vi "spindle_speed_1.vi"(0 "Byte Stream File in":refnum<file>, 2 "Array":dbl[](array[numeric]), 5 "base path":path, 7 "Record  SS 661":bool, 9 "Boolean 3":bool, 11 "error in (no error)":errorcluster, 12 "Initial Time in":timestamp, 13 "Stop Program 4":bool) -> (4 "Byte Stream File out":refnum<file>, 6 "Boolean 2":bool, 8 "Initial Time out":timestamp, 10 "Stop Program 5":bool, 15 "error out":errorcluster)   [LabVIEW 2014]
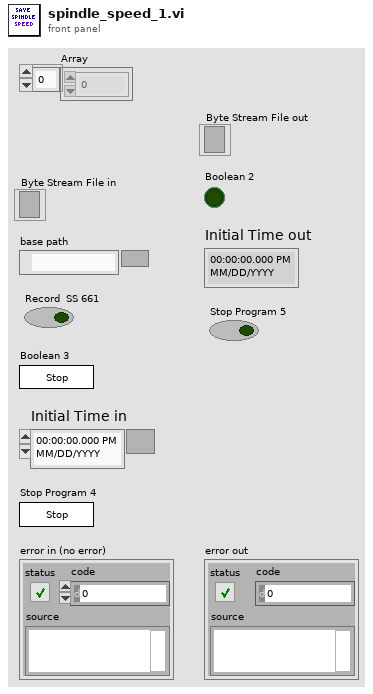
[diagram p1: front panel]
types:
  T1 = cluster{"Array":dbl[], "seconds since 1Jan1904":timestamp}
  T2 = enum16{"NotSaving", "Create", "Reading", "Closing"}
  T3 = enum16{"open", "replace", "create", "open or create", "replace or create", "replace or create with confirmation"}
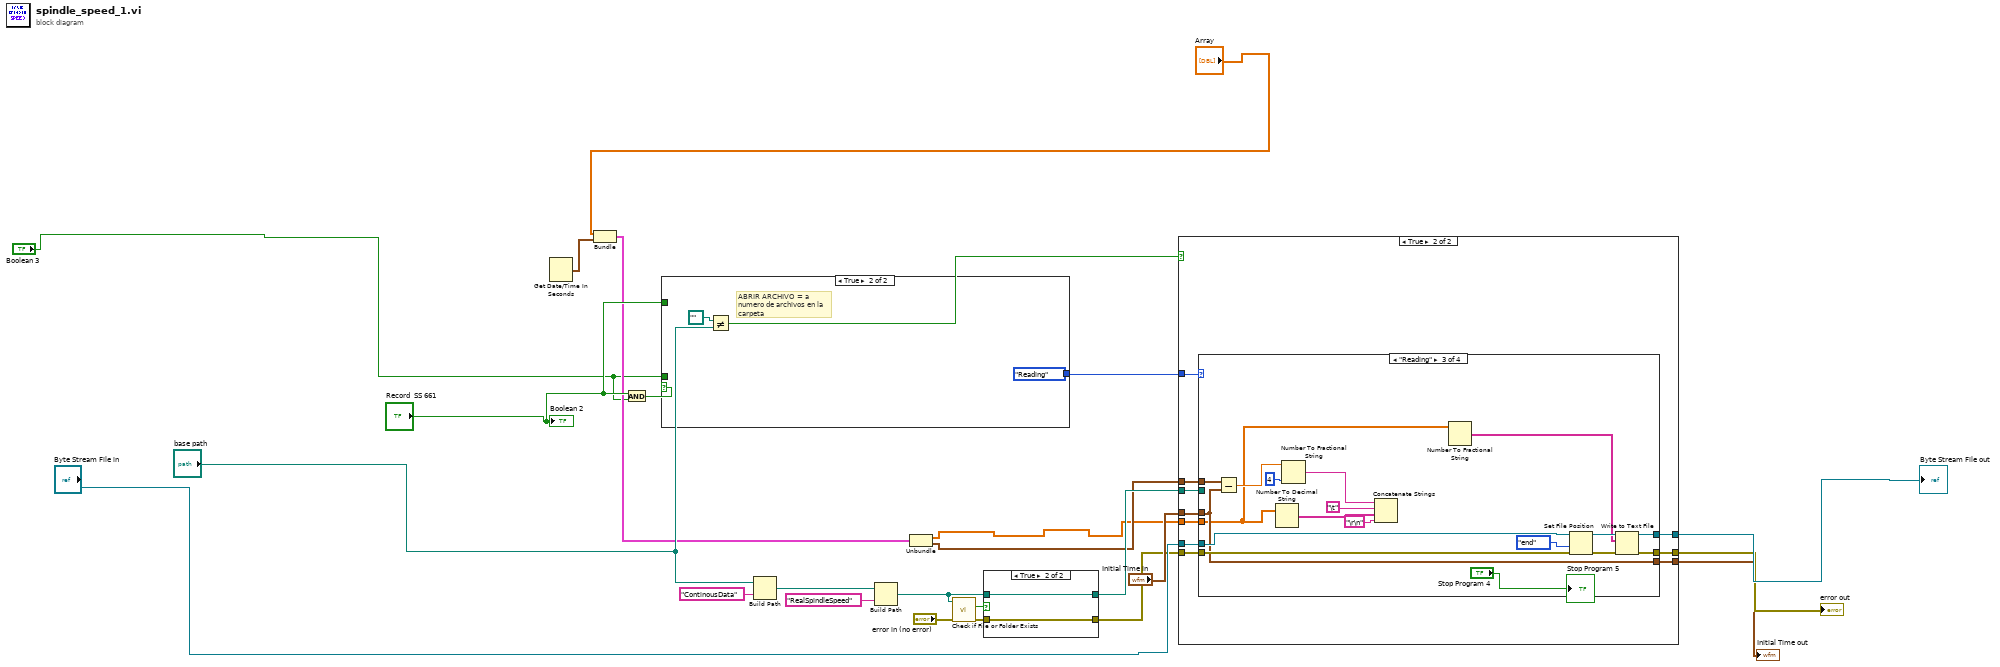
[diagram p0: block diagram]
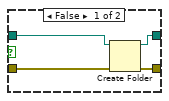
[diagram p2: hidden frame]
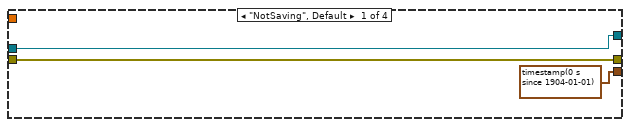
[diagram p4: hidden frame]
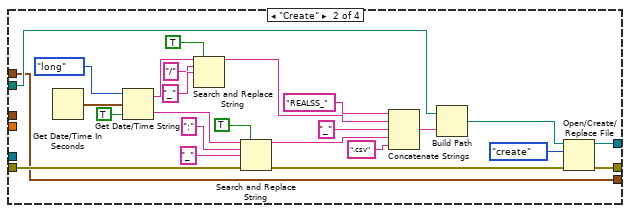
[diagram p5: hidden frame]
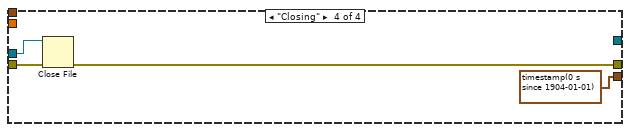
[diagram p6: hidden frame]
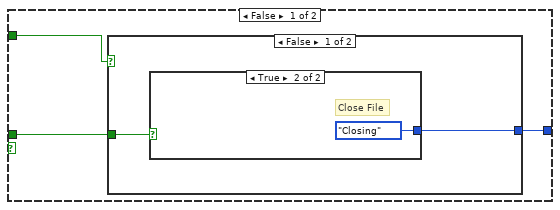
[diagram p7: hidden frame]
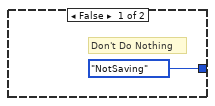
[diagram p8: hidden frame]
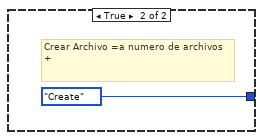
[diagram p9: hidden frame]
diagram:
  n1 = Get Date/Time In Seconds() -> (seconds since 1Jan1904=w6:timestamp)
  n2 = Bundle("Array"="Array", "seconds since 1Jan1904"=w6) -> (w5:T1)  [unwired: 1 in]
  n3 = And(x="Record  SS 661", y="Boolean 3") -> (x .and. y?=w21:bool)
  n4 = case shown="True" w21 {
    tunnel: "Boolean 3" -> [w30 _]
    tunnel: [w29 T2."Reading" ("Enum")] -> w20
    tunnel: "Record  SS 661" -> [w28 _]
    frame False {
      n5 = case shown="False" w28 {
        tunnel: w30 -> [w32 _]
        tunnel: [w31 T2."Create" ("Enum")] -> w29
        frame False {
          n6 = case shown="True" w32 {
            tunnel: [T2."NotSaving" ("Enum") T2."Closing" ("Enum")] -> w31
            frame False {
              # "Don't Do Nothing"
            }
            frame True {
              # "Close File"
            }
          }
        }
        frame True {
          # "Crear Archivo =a numero de archivos +"
        }
      }
    }
    frame True {
      # "ABRIR ARCHIVO = a numero de archivos en la carpeta"
    }
  }
  n7 = Not Equal?(x=path "" ("Project Folder"), y="base path") -> (x != y?=w14:bool)
  n8 = Build Path(base path="base path", name or relative path="ContinousData") -> (appended path=w10:path)
  n9 = Build Path(base path=w10, name or relative path="RealSpindleSpeed") -> (appended path=w9:path)
  n10 = Unbundle(w5) -> ("Array"=w3:dbl[], "seconds since 1Jan1904"=w4:timestamp)
  n11 = call <vilib>:"Check if File or Folder Exists.vi"("error in (no error)"="error in (no error)", "path"=w9) -> ("error out"=w12:errorcluster, "file or folder exists?"=w13:bool)  [unwired: 7 in, 1 out]
  n12 = case shown="True" w13 {
    tunnel: [w40 w42] -> w7
    tunnel: w12 -> [w39 w42]
    tunnel: w9 -> [w38 w41]
    tunnel: [w37 w41] -> w8
    frame False {
      n13 = Create Folder(path (use dialog)=w38, error in=w39) -> (created path=w37:path, error out=w40:errorcluster)  [unwired: 1 in, 1 out]
    }
    frame True {
    }
  }
  n14 = case shown="True" w14 {
    tunnel: w8 -> [_ w51]
    tunnel: w3 -> [_ w53]
    tunnel: w20 -> [_ w52]
    tunnel: w7 -> [w43 w50]
    tunnel: "Byte Stream File in" -> [_ w49]
    tunnel: [_ w48] -> w26
    tunnel: [w43 w47] -> w19
    tunnel: [_ w46] -> w18
    tunnel: "Initial Time in" -> [_ w45]
    tunnel: w4 -> [_ w44]
    frame False {
    }
    frame True {
      n15 = case shown="\"Reading\"" w52 {
        tunnel: w53 -> [_ _ w83 _]
        tunnel: w51 -> [_ w81 _ _]
        tunnel: w50 -> [w56 w62 w94 w102]
        tunnel: w49 -> [w55 _ w97 w100]
        tunnel: [w55 w60 w90 _] -> w48
        tunnel: [w56 w59 w91 w101] -> w47
        tunnel: [timestamp(0 s since 1904-01-01) ("Initial Time") w57 w89 timestamp(0 s since 1904-01-01) ("Initial Time")] -> w46
        tunnel: w45 -> [_ _ w89 _]
        tunnel: w44 -> [_ w57 w88 _]
        frame "NotSaving", Default {
        }
        frame "Create" {
          n16 = Get Date/Time In Seconds() -> (seconds since 1Jan1904=w78:timestamp)
          n17 = Get Date/Time String(date format (0)=enum16{"short", "long", "abbreviated"}."long", seconds (now)=w78, want seconds? (F)=TRUE) -> (date string=w76:string, time string=w72:string)
          n18 = Search and Replace String(replace all?=TRUE ("replace all? (F)"), input string=w76, search string="/", replace string="_" ("replace string (\"\")")) -> (result string=w69:string)  [unwired: 4 in, 3 out]
          n19 = Search and Replace String(replace all?=TRUE ("replace all? (F)"), input string=w72, search string=":", replace string="_" ("replace string (\"\")"), error in=w62) -> (result string=w67:string, error out=w63:errorcluster)  [unwired: 3 in, 2 out]
          n20 = Concatenate Strings("REALSS_" ("string"), w69, "_" ("string"), w67, ".csv" ("string")) -> (w65:string)
          n21 = Build Path(base path=w81, name or relative path=w65) -> (appended path=w80:path)
          n22 = Open/Create/Replace File(file path (use dialog)=w80, error in=w63, operation (0:open)=T3."create") -> (refnum out=w60:refnum<file>, error out=w59:errorcluster)  [unwired: 3 in, 1 out]
        }
        frame "Reading" {
          n23 = Subtract(x=w88, y=w89) -> (x-y=w86:dbl)
          n24 = Number To Decimal String(number=w83) -> (decimal integer string=w93:string[])  [unwired: 1 in]
          n25 = Number To Fractional String(number=w86, precision (6)=i16 4) -> (F-format string=w84:string)  [unwired: 2 in]
          n26 = Concatenate Strings(w84, "\t", w93, "\r\n") -> ()  [unwired: 1 out]
          n27 = Number To Fractional String(number=w83) -> (F-format string=w82:string[])  [unwired: 3 in]
          n28 = Set File Position(refnum=w97, from (0:start)=enum16{"start", "end", "current"}."end", error in=w94) -> (refnum out=w96:refnum<file>, error out=w95:errorcluster)  [unwired: 1 in]
          n29 = Write to Text File(file (use dialog)=w96, text=w82, error in=w95) -> (refnum out=w90:refnum<file>, error out=w91:errorcluster)  [unwired: 1 in, 1 out]
        }
        frame "Closing" {
          n30 = Close File(refnum=w100, error in=w102) -> (error out=w101:errorcluster)  [unwired: 1 out]
        }
      }
    }
  }
  "error out" <- w19
  "Initial Time out" <- w18
  "Byte Stream File out" <- w26
  "Boolean 2" <- "Record  SS 661"
  "Stop Program 5" <- "Stop Program 4"
